vi "Open COM Port.vi"(8 "error in (no error)":errorcluster, 11 "Abstract Spectrometer in":refnum<class "Abstract Spectrometer.lvclass">) -> (0 "error out":errorcluster, 3 "Abstract Spectrometer out":refnum<class "Abstract Spectrometer.lvclass">)   [LabVIEW 2019, in "Spectrometer.lvlib"]
uses:
  Spectrometer.lvlib
  Spectrometer-LVClass/Abstract Spectrometer_class/Abstract Spectrometer.lvclass
  <vilib>/Utility/config.llb/Read Key (String).vi
  <vilib>/Utility/config.llb/NI_LVConfig.lvlib
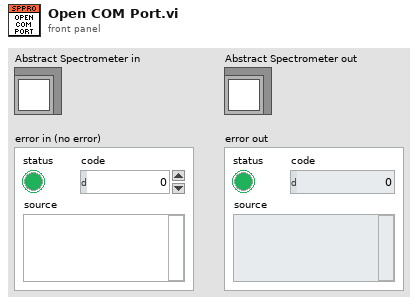
[diagram p1: front panel]
types:
  T1 = typedef "NI_LVConfig.lvlib/Config Data RefNum.ctl" = refnum<k1>
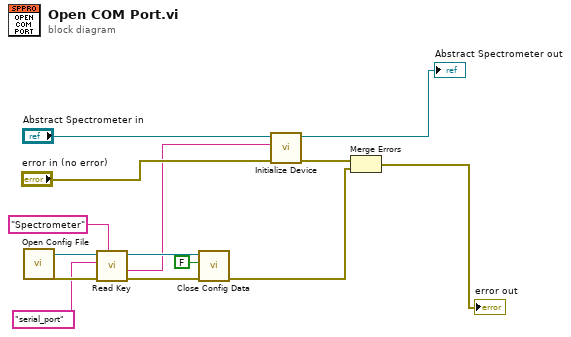
[diagram p0: block diagram]
diagram:
  n1 = call "Open Config File.vi"() -> ("error out"=w9:errorcluster, "Refnum out"=w8:T1)  [unwired: 10 in]
  n2 = call-poly <vilib>:"Read Key.vi"("section"="Spectrometer", "error in (no error)"=w9, "key"="serial_port", "refnum"=w8) -> ("error out"=w7:errorcluster, "value"=w3:string, "refnum out"=w6:T1)  [unwired: 4 in, 1 out]
  n3 = call <vilib>:"Close Config Data.vi"("error in (no error)"=w7, "write file if changed (T)"=FALSE, "refnum"=w6) -> ("error out"=w4:errorcluster)  [unwired: 7 in, 1 out]
  n4 = call-dynamic "Initialize Device.vi"("error in (no error)"="error in (no error)", "VISA resource name"=w3, "Abstract Spectrometer in"="Abstract Spectrometer in") -> ("error out"=w12:errorcluster, "Abstract Spectrometer out"=→"Abstract Spectrometer out":refnum<class "Abstract Spectrometer.lvclass">)  [unwired: 7 in]
  n5 = Merge Errors(w12, w4) -> (→"error out":errorcluster)
